vi "Get User Interface VI.vi"(8 "error in":errorcluster, 11 "RDMA Transfer Tx User Interface in":refnum<class "RDMA Transfer Tx User Interface.lvclass">) -> (0 "error out":errorcluster, 2 "user interface vi":refnum<vi>, 3 "RDMA Transfer Tx User Interface out":refnum<class "RDMA Transfer Tx User Interface.lvclass">)   [LabVIEW 2020, in "RDMA.lvlib" / "RDMA Transfer Tx User Interface.lvclass"]
uses:
  RDMA Transfer Tx User Interface.lvclass
  User Interface.vi
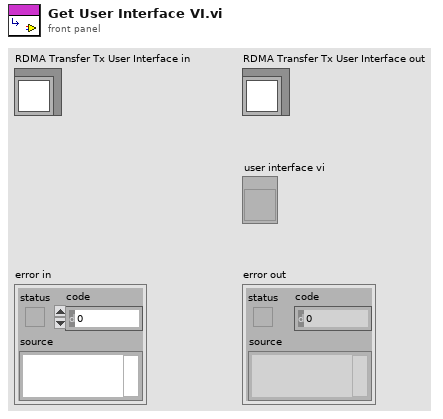
[diagram p1: front panel]
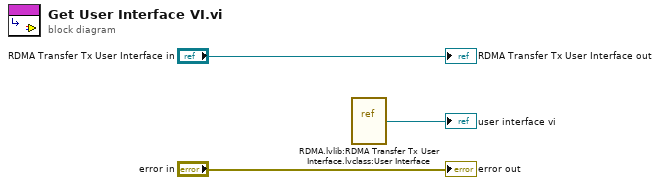
[diagram p0: block diagram]
diagram:
  n1 = vi-ref "RDMA.lvlib:RDMA Transfer Tx User Interface.lvclass:User Interface.vi"() -> (→"user interface vi":refnum<vi>)
  "error out" <- "error in"
  "RDMA Transfer Tx User Interface out" <- "RDMA Transfer Tx User Interface in"
